vi "BRig_Host_dataRunState_dataTS_tSelection.vi"() -> (2 "output_idx_dataTS_tSelection":i32)   [LabVIEW 2014]
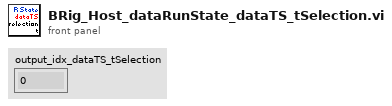
[diagram p1: front panel]
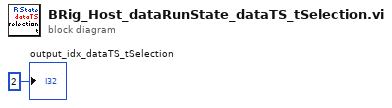
[diagram p0: block diagram]
diagram:
  "output_idx_dataTS_tSelection" <- 2 ("output_idx_dataTS")
